vi "ERDWrite_To_GEA2.vi"() -> ()   [LabVIEW 2014]
uses:
  type defs/ERD Write Data In.ctl
  type defs/Source_Destination.ctl
  type defs/Data In.ctl
  library/GEA2_Toolkit.lvlib
panel:
  out "Error Out":errorcluster
  in  "Error In":errorcluster
  out "GEA2 Message Data":T1 {"Command" format="%02x"; "Destination" format="%02x"; "Source" format="%02x"}
  in  "GEA Inputs":T2 {"Destination" format="%.0x"; "Source" format="%.0x"}
  in  "Write ERD List":T3[](array[typedef]) {"ERD Number" format="%.0x"}
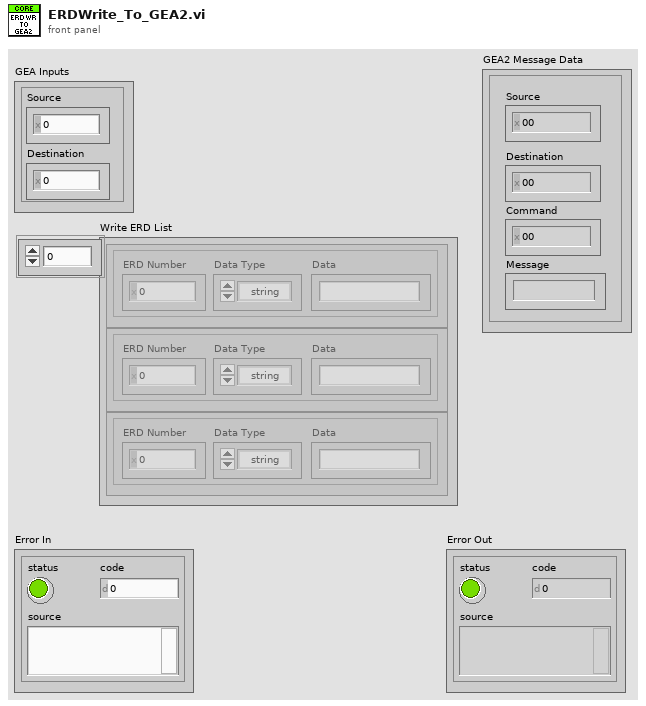
[diagram p1: front panel]
types:
  T1 = typedef "GEA2_Toolkit.lvlib/Data In.ctl" = cluster{"Source":u8, "Destination":u8, "Command":u8, "Message":string}
  T2 = typedef "GEA2_Toolkit.lvlib/Source_Destination.ctl" = cluster{"Source":u8, "Destination":u8}
  T3 = typedef "GEA2_Toolkit.lvlib/ERD Write Data In.ctl" = cluster{"ERD Number":u16, "Data Type":enum16{"string", "boolean", "uint8_t", "uint16_t", "uint32_t"}, "Data":string}
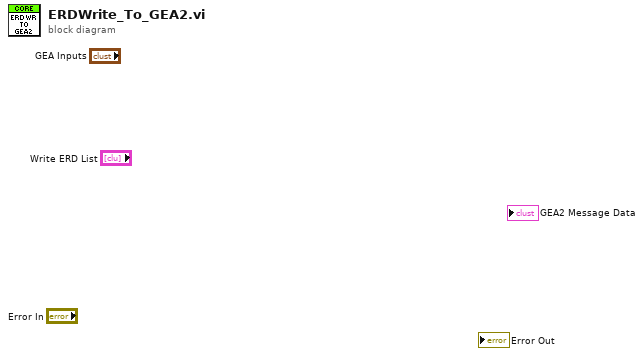
[diagram p0: block diagram]
diagram:
